vi "数值转换.vi"(11 "数组":u16[](array[numeric])) -> (3 "显示值":T1)   [LabVIEW 2016, in "流量计集成.lvlib" / "流量计.lvlib"]
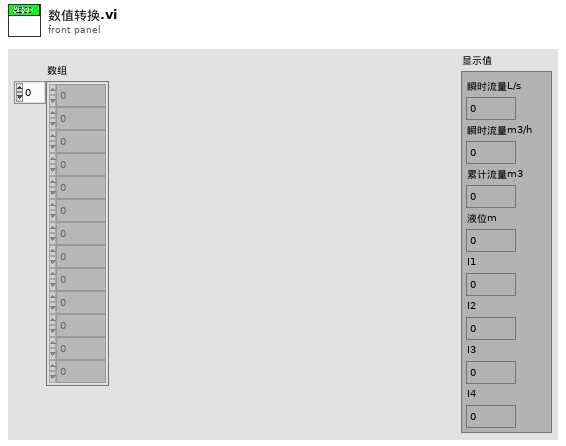
[diagram p1: front panel]
types:
  T1 = cluster{"瞬时流量L/s":dbl, "瞬时流量m3/h":dbl, "累计流量m3":dbl, "液位m":dbl, "I1":dbl, "I2":dbl, "I3":dbl, "I4":dbl}
  T2 = cluster{"[0]":sgl, "[1]":sgl, "[2]":sgl, "[3]":sgl, "[4]":sgl, "[5]":sgl, "[6]":sgl, "[7]":sgl}
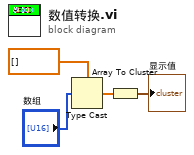
[diagram p0: block diagram]
diagram:
  n1 = Type Cast(type=sgl[] [], x="数组") -> (*(type *) &x=w2:sgl[])
  n2 = Array To Cluster(array=w2) -> (cluster=→"显示值":T2)
